vi "Request Current State.vi"(8 "error in (no error)":errorcluster, 9 "Requestor Queue":refnum<class "Message Enqueuer.lvclass">, 10 "Elevator.lvlib:Current State Msg.lvclass":refnum<class "Current State Msg.lvclass">, 11 "Elevator in":refnum<class "Elevator.lvclass">) -> (0 "error out":errorcluster, 3 "Elevator out":refnum<class "Elevator.lvclass">)   [LabVIEW 2014, in "Elevator.lvlib" / "Elevator.lvclass"]
uses:
  Elevator.lvclass
  Elevator Messages/Current State Msg/Current State Msg.lvclass
  <vilib>/ActorFramework/Message Enqueuer/Message Enqueuer.lvclass
  Elevator Messages/Current Motors with Encoder State Msg/Current Motors with Encoder State Msg.lvclass
  <vilib>/ActorFramework/Actor/Actor.lvclass/Actor.ctl
  <vilib>/ActorFramework/Message Enqueuer/Message Enqueuer.lvclass/Message Enqueuer.ctl
  Elevator.lvclass/Elevator.ctl
  Motor with Encoders/Motors with Encoders Messages/Request Motors with Encoders State Msg/Request Motors with Encoders State Msg.lvclass/Request Motors with Encoders State Msg.ctl
  Elevator Messages/Current State Msg/Current State Msg.lvclass/Current State Msg.ctl
  <vilib>/ActorFramework/Message Enqueuer/Init from Existing Queue.vi
  <vilib>/ActorFramework/Message Enqueuer/Enqueue.vi
  <vilib>/ActorFramework/Message Priority Queue/Priority Enqueue.vi
  Motor with Encoders/Motors with Encoders Messages/Request Motors with Encoders State Msg/Request Motors with Encoders State Msg.lvclass
  <vilib>/ActorFramework/Actor/Actor.lvclass
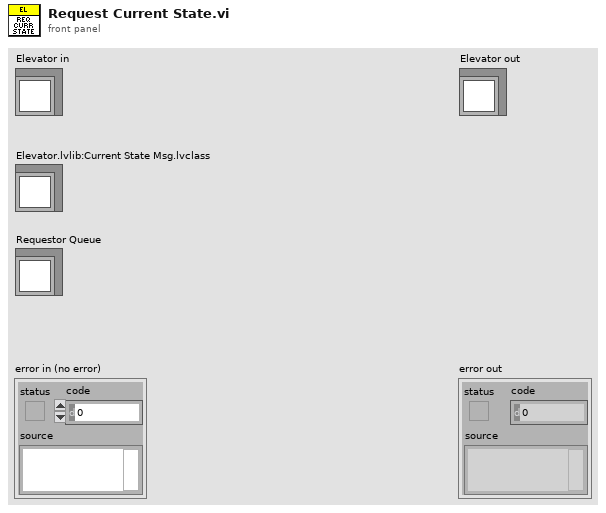
[diagram p1: front panel]
types:
  T1 = typedef "Elevator.lvlib/Elevator.lvclass/Elevator State.ctl" = cluster{"At Bottom":bool, "At Top":bool, "At Setpoint":bool, "Target Rate (RPM)":dbl, "Current Travel Rate":dbl, "Current Elevation":dbl, "Brake On":bool, "Motor Elevate Rate (RPM))":dbl, "Has Been Home":bool}
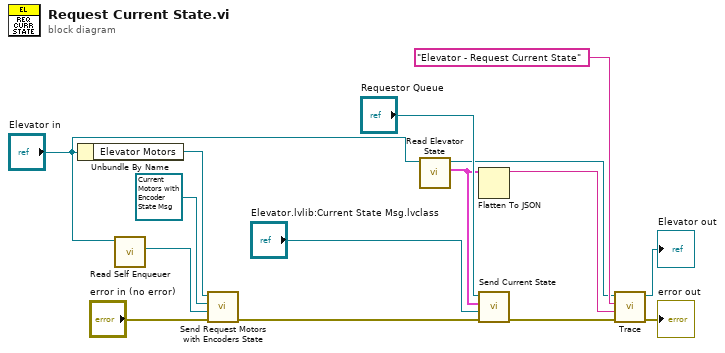
[diagram p0: block diagram]
diagram:
  n1 = Unbundle By Name("Elevator in") -> ("Elevator Motors"=w15:refnum<class "Message Enqueuer.lvclass">)
  n2 = call <vilib>:"Read Self Enqueuer.vi"("Actor"="Elevator in") -> ("Self Enqueuer"=w10:refnum<class "Message Enqueuer.lvclass">)  [unwired: 10 in]
  n3 = call "Send Request Motors with Encoders State.vi"("error in (no error)"="error in (no error)", "Requestor Queue"=w10, "Current State Msg"=refnum<class "Current Motors with Encoder State Msg.lvclass"> refnum ("Elevator.lvlib:Current Motors with Encoder State Msg.lvclass"), "Message Enqueuer"=w15) -> ("error out"=w4:errorcluster)  [unwired: 6 in, 1 out]
  n4 = call-dynamic "Read Elevator State.vi"("Elevator in"="Elevator in") -> ("Elevator State"=w2:T1, "Elevator out"=w1:refnum<class "Elevator.lvclass">)  [unwired: 8 in, 1 out]
  n5 = Flatten To JSON(anything=w2) -> (JSON string=w9:string)  [unwired: 2 in, 1 out]
  n6 = call "Send Current State.vi"("error in (no error)"=w4, "Elevator.lvlib:Current State Msg.lvclass"="Elevator.lvlib:Current State Msg.lvclass", "Elevator State"=w2, "Message Enqueuer"="Requestor Queue") -> ("error out"=w7:errorcluster)  [unwired: 6 in, 1 out]
  n7 = call-dynamic "Trace.vi"("error in (no error)"=w7, "System Message"=w9, "System Action"="Elevator - Request Current State", "System Actor in"=w1) -> ("error out"=→"error out":errorcluster, "System Actor out"=→"Elevator out":refnum<class "Elevator.lvclass">)  [unwired: 6 in]
